vi "sort unknowns from stds.vi"(8 "error in":errorcluster) -> (0 "error out":errorcluster, 3 "output cluster":T1 {"cycle results dbl" format="%#_11f"})   [LabVIEW 2016]
uses:
  controls/cycle results control.ctl
panel:
  out "cycle results cluster result":T1 {"cycle results dbl" format="%#_6e"}
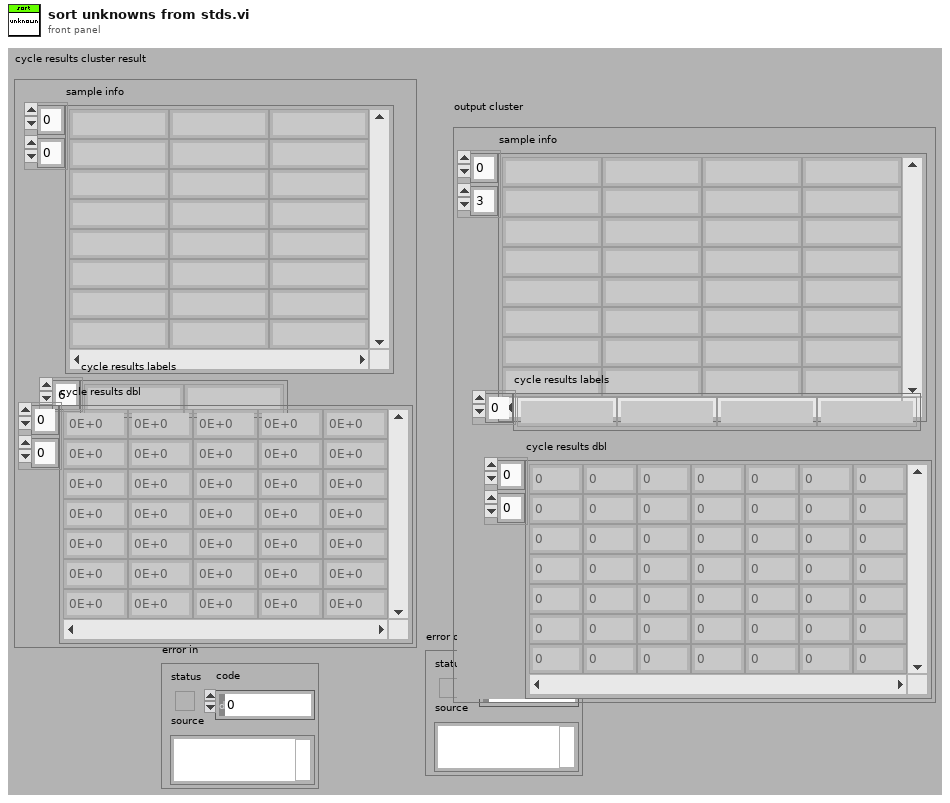
[diagram p1: front panel]
types:
  T1 = typedef "cycle results control.ctl" = cluster{"sample info":string[][], "cycle results labels":string[], "cycle results dbl":dbl[][]}
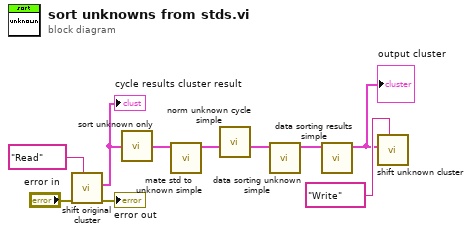
[diagram p0: block diagram]
diagram:
  n1 = call "shift original cluster.vi"("read write shift"="Read", "error in"="error in") -> ("error out"=→"error out":errorcluster, "cycle results cluster out"=w8:T1)  [unwired: 8 in]
  "cycle results cluster result" <- w8
  n2 = call "sort unknown only.vi"("cycle results cluster out  2"=w8) -> ("cycle results cluster out"=w5:T1)
  n3 = call "mate std to unknown simple.vi"("cycle results cluster result"=w5) -> ("output cluster"=w4:T1)  [unwired: 9 in, 1 out]
  n4 = call "norm unknown cycle simple.vi"("output cluster 2"=w4) -> ("output cluster"=w3:T1)  [unwired: 10 in]
  n5 = call "data sorting unknown simple.vi"("cycle results cluster IN"=w3) -> ("cycle results cluster out"=w2:T1)  [unwired: 9 in, 1 out]
  n6 = call "data sorting results simple.vi"("cycle results cluster IN"=w2) -> ("cycle results cluster out"=w1:T1)  [unwired: 9 in, 1 out]
  "output cluster" <- w1
  n7 = call "shift unknown cluster.vi"("read write shift"="Write", "cycle results cluster In"=w1) -> ()  [unwired: 8 in, 2 out]
